vi "Get WIFI Secuirty Type.vi"(8 "Error In":errorcluster, 11 "LINX Device Config":T2) -> (0 "Error Out":errorcluster, 3 "LINX Device Config":T2, 10 "WIFI Security Type":T1=enum."WPA2 Password")   [LabVIEW 2011, in "LVH-LINX.lvlib" / "Device.lvlib"]
doc: "Get the LINX device's WIFI Security Type."
uses:
  Device.lvlib
  Type Defs/LINX Device Config.ctl
  Type Defs/Interface.ctl
  Type Defs/TCP Config.ctl
  Type Defs/Channels.ctl
  Type Defs/WIFI Security Type.ctl
  Type Defs/Error Type.ctl
  LVH-LINX.lvlib
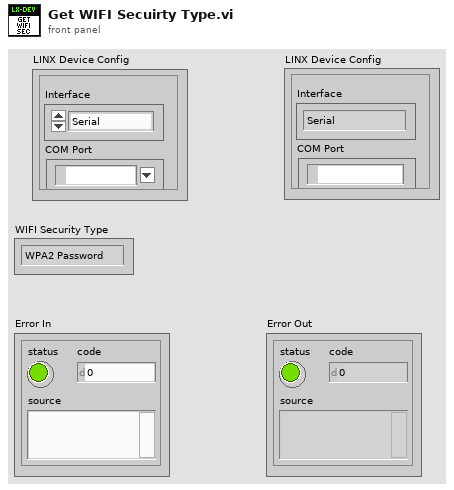
[diagram p1: front panel]
types:
  T1 = typedef "LVH-LINX.lvlib/WIFI Security Type.ctl" = enum8{"None", "WPA2 Password", "WPA2 Key", "WEP40", "WEP104"}
  T2 = typedef "LVH-LINX.lvlib/Device.lvlib/LINX Device Config.ctl" = cluster{"Interface":T3, "COM Port":refnum<visa-resource-name>, "TCP Configuration":T4, "Device Family":u8, "Device ID":u8, "Device Name":string, "TCP Ref":refnum<k5>, "Channels":T5}
  T3 = typedef "LVH-LINX.lvlib/Interface.ctl" = enum16{"Serial", "TCP"}
  T4 = typedef "LVH-LINX.lvlib/Device.lvlib/TCP Config.ctl" = cluster{"IP Address":string, "Port":u16}
  T5 = typedef "LVH-LINX.lvlib/Channels.ctl" = cluster{"DI Channels":u8[], "DO Channels":u8[], "AI":u8[], "AO":u8[], "PWM":u8[], "QE":u8[], "UART":u8[], "I2C 2":u8[], "SPI":u8[], "CAN":u8[], "AI Ref (V)":dbl, "AO Resolution (Bits)":u8, "AO Ref (V)":dbl}
  T6 = typedef "LVH-LINX.lvlib/Error Type.ctl" = enum16{"Unknown", "Timeout", "Corrupt Return Packet", "Unable To Connect", "Command Not Supported", "Channel DNE", "Invalid COM Config", "Firmware Version Mismatch", "myRIO Support"}
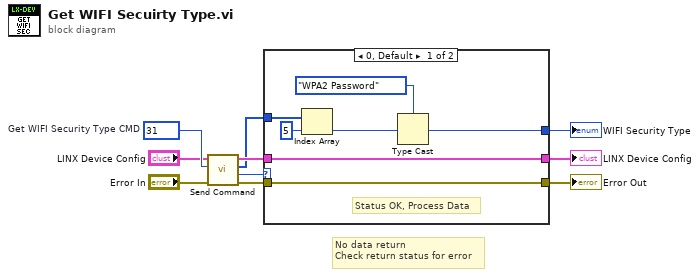
[diagram p0: block diagram]
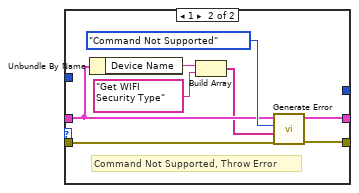
[diagram p2: hidden frame]
diagram:
  w9 = u16 31  # Get WIFI Security Type CMD
  # "No data return\nCheck return status for error"
  n1 = call "Send Command.vi"("Error In"="Error In", "CMD"=w9, "LINX Device Config"="LINX Device Config") -> ("Error Out"=w4:errorcluster, "Status"=w2:u8, "Response"=w3:u8[], "LINX Device Config"=w6:T2)  [unwired: 5 in]
  n2 = case shown="0, Default" w2 {
    tunnel: [w16 w23] -> w7
    tunnel: w6 -> [w16 w19]
    tunnel: [w17 w24] -> w5
    tunnel: w4 -> [w17 w25]
    tunnel: w3 -> [w15 _]
    tunnel: [w11 _] -> w1
    frame 0, Default {
      # "Status OK, Process Data"
      n3 = Index Array(array=w15, index=5) -> (element=w13:u8)
      n4 = Type Cast(type=WIFI_Security_Type."WPA2 Password" ("WIFI Security Type"), x=w13) -> (*(type *) &x=w11:T1)
    }
    frame 1 {
      # "Command Not Supported, Throw Error"
      n5 = Unbundle By Name(w19) -> ("Device Name"=w20:string)
      n6 = Build Array(w20, "Get WIFI Security Type") -> (w18:string[])
      n7 = call "Generate Error.vi"("Error In"=w25, "Arguments"=w18, "Error Type"=Error_Type."Command Not Supported", "LINX Device Config"=w19) -> ("Error Out"=w24:errorcluster, "LINX Device Config"=w23:T2)  [unwired: 6 in]
    }
  }
  "Error Out" <- w5
  "LINX Device Config" <- w7
  "WIFI Security Type" <- w1
